vi "SW_Load_data_from_older_TDMS.vi"(4 "Data samples to load":i64=-1, 8 "error in (no error)":errorcluster, 11 "TDMS file ref.":refnum<k34>) -> (0 "error out":errorcluster, 1 "Start time":dbl, 2 "Author's name":string, 3 "Loaded data":T1={"Absolute timestamp (DBL)"=[], "Relative timestamp (DBL)"=[], "Zones normalized allocation array"=[], "Coordinates and speed"=[], "Current zone and TTLs"=[], "Acquisition settings cluster out"={"Researcher name"="", "N segments MIDFIELD"=0, "N segments BORDER"=0, "Radius, mm CENTER"=0, "Radius, mm MIDFIELD"=0, "Starting angle MIDFIELD"=0, "Starting angle BORDER"=0, "Cage diameter, mm"=0, "Bridge swap"=FALSE, "Bridge V. offset"=0.0, "Twisted neck"=FALSE, "Offset H."=0.0, "Name prefix"="SavedTrack", "Stop at"=0.0, "\"Stop at\" enabled"=FALSE, "Settings loaded OK"=FALSE}, "Stimulus presets array"=[]} {"Acquisition settings cluster out"."Stop at" format="%<%H:%M:%S>t"}, 5 "Data loaded OK":bool, 7 "Settings loaded OK":bool)   [LabVIEW 2018, in "Tracker.lvlib"]
uses:
  Tracker.lvlib
panel:
  out "Stimulus presets array (loaded)":T2(array[cluster])
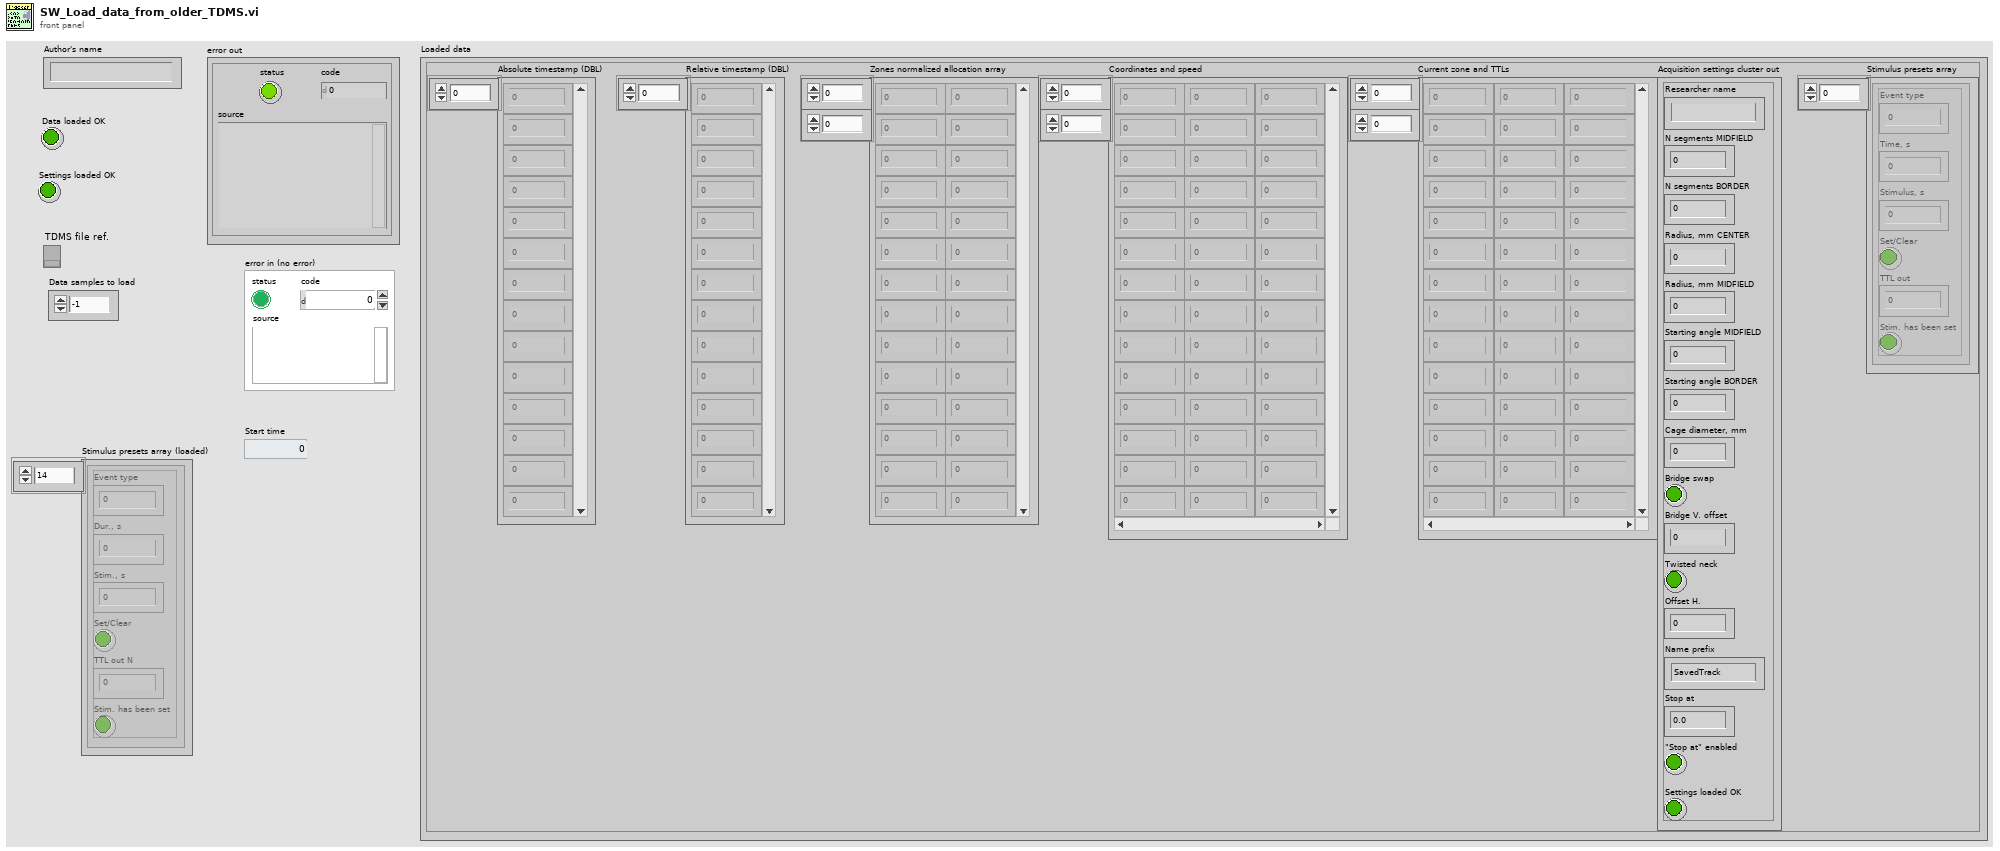
[diagram p1: front panel]
types:
  T1 = cluster{"Absolute timestamp (DBL)":dbl[], "Relative timestamp (DBL)":dbl[], "Zones normalized allocation array":dbl[][], "Coordinates and speed":dbl[][], "Current zone and TTLs":u8[][], "Acquisition settings cluster out":cluster{"Researcher name":string, "N segments MIDFIELD":u8, "N segments BORDER":u8, "Radius, mm CENTER":u16, "Radius, mm MIDFIELD":u16, "Starting angle MIDFIELD":i16, "Starting angle BORDER":i16, "Cage diameter, mm":u16, "Bridge swap":bool, "Bridge V. offset":sgl, "Twisted neck":bool, "Offset H.":sgl, "Name prefix":string, "Stop at":dbl, "\"Stop at\" enabled":bool, "Settings loaded OK":bool}, "Stimulus presets array":cluster{"Event type":u16, "Time, s":sgl, "Stimulus, s":sgl, "Set/Clear":bool, "TTL out":u16, "Stim. has been set":bool}[]}
  T2 = cluster{"Event type":u16, "Dur., s":sgl, "Stim., s":sgl, "Set/Clear":bool, "TTL out N":u16, "Stim. has been set":bool}[]
  T3 = cluster{"N segments BORDER":u8, "Starting angle BORDER":i16, "N segments MIDFIELD":u8, "Starting angle MIDFIELD":i16, "Radius, mm MIDFIELD":u16, "Amount of central segments":u8, "Radius, mm CENTER":u16, "Bridge swap":bool, "Bridge V. offset":sgl, "Twisted neck":bool, "Offset H.":sgl, "Zones configuration":string[], "IO parameters string":string, "Cage diameter, mm":u16, "Name prefix":string, "Stop at":dbl, "\"Stop at\" enabled":bool}
  T4 = cluster{"Event type":u16, "Time, s":sgl, "Stimulus, s":sgl, "Set/Clear":bool, "TTL out":u16, "Stim. has been set":bool}
  T5 = cluster{string, "N segments MIDFIELD":u8, "N segments BORDER":u8, "Radius, mm CENTER":u16, "Radius, mm MIDFIELD":u16, "Starting angle MIDFIELD":i16, "Starting angle BORDER":i16, "Cage diameter, mm":u16, "Bridge swap":bool, "Bridge V. offset":sgl, "Twisted neck":bool, "Offset H.":sgl, "Name prefix":string, "Stop at":dbl, "\"Stop at\" enabled":bool, bool}
  T6 = cluster{dbl[], dbl[], "Zones normalized allocation array":dbl[][], dbl[][], u8[][], cluster{string, "N segments MIDFIELD":u8, "N segments BORDER":u8, "Radius, mm CENTER":u16, "Radius, mm MIDFIELD":u16, "Starting angle MIDFIELD":i16, "Starting angle BORDER":i16, "Cage diameter, mm":u16, "Bridge swap":bool, "Bridge V. offset":sgl, "Twisted neck":bool, "Offset H.":sgl, "Name prefix":string, "Stop at":dbl, "\"Stop at\" enabled":bool, bool}, cluster{"Event type":u16, "Time, s":sgl, "Stimulus, s":sgl, "Set/Clear":bool, "TTL out":u16, "Stim. has been set":bool}[]}
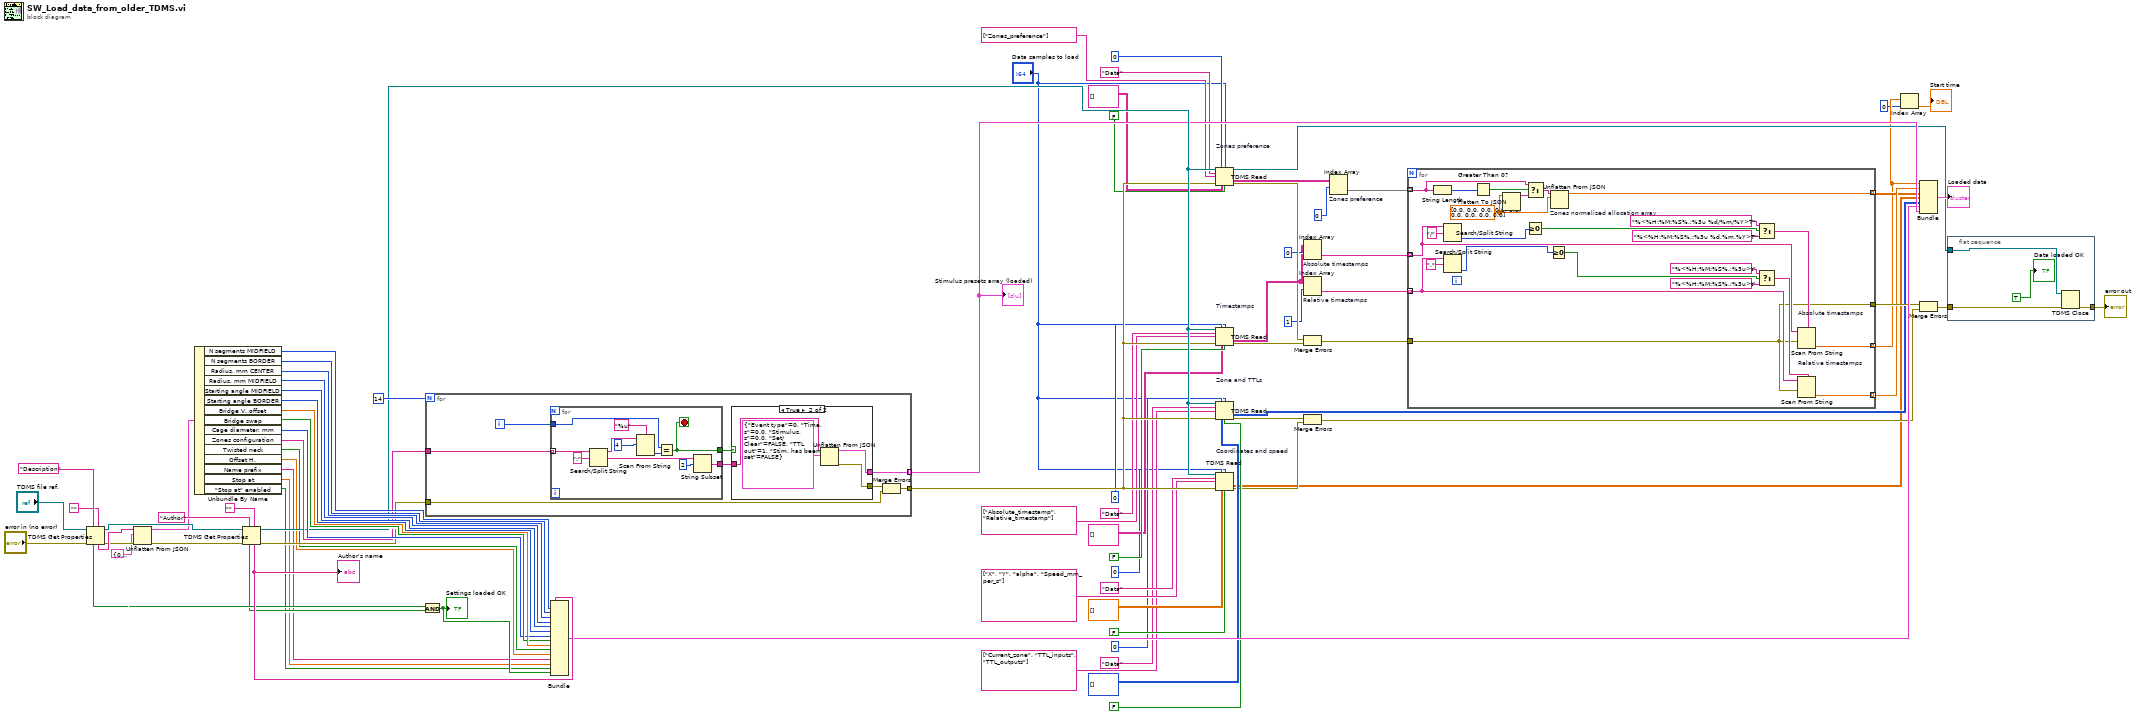
[diagram p0: block diagram]
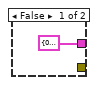
[diagram p2: hidden frame]
diagram:
  n1 = TDMS Get Properties(5:"", 7:"Description" ("property name"), 8:"error in (no error)", 11:"TDMS file ref.") -> (0:w81:errorcluster, 3:w80:refnum<k34>, 4:w82:string, 6:w65:bool)  [unwired: 2 in, 2 out]
  n2 = Unflatten From JSON(JSON string=w82, type and defaults=T3 {"N segments BORDER"=0, "Starting angle BORDER"=0, "N segments MIDFIELD"=0, "Starting angle MIDFIELD"=0, "Radius, mm MIDFIELD"=0, "Amount of central segments"=0, "Radius, mm CENTER"=0, "Bridge swap"=FALSE, "Bridge V. offset"=0.0, "Twisted neck"=FALSE, "Offset H."=0.0, "Zones configuration"=[], "IO parameters string"="[12,1,1,0,0,0]", "Cage diameter, mm"=180, "Name prefix"="SavedTrack", "Stop at"=0.0, "\"Stop at\" enabled"=FALSE} ("Parameters"), error in (no error)=w81) -> (value=w67:T3, error out=w77:errorcluster)  [unwired: 4 in]
  n3 = Unbundle By Name(w67) -> ("N segments MIDFIELD"=w75:u8, "N segments BORDER"=w74:u8, "Radius, mm CENTER"=w73:u16, "Radius, mm MIDFIELD"=w72:u16, "Starting angle MIDFIELD"=w71:i16, "Starting angle BORDER"=w70:i16, "Bridge V. offset"=w69:sgl, "Bridge swap"=w68:bool, "Cage diameter, mm"=w66:u16, "Zones configuration"=w62:string[], "Twisted neck"=w54:bool, "Offset H."=w53:sgl, "Name prefix"=w52:string, "Stop at"=w51:dbl, "\"Stop at\" enabled"=w50:bool)
  n4 = TDMS Get Properties(5:"", 7:"Author" ("property name"), 8:w77, 11:w80) -> (0:w63:errorcluster, 3:w60:refnum<k34>, 4:w76:string, 6:w64:bool)  [unwired: 2 in, 2 out]
  "Author's name" <- w76
  n5 = And(x=w65, y=w64) -> (x .and. y?=w55:bool)
  "Settings loaded OK" <- w55
  n6 = for {
    N: 14 -> [_]
    tunnel: w63 -> [w89]
    tunnel: [w91] -> w59
    tunnel: [w92] -> w58 mode=indexing
    tunnel: w62 -> [w87]
    i -> [w88]
    n7 = for {
      tunnel: w87 -> [w103] mode=indexing
      tunnel: w88 -> [w97]
      tunnel: [w96] -> w86
      tunnel: [w95] -> w85
      stop <- w96 stop-if-true
      n8 = Search/Split String(string=w103, search string/char (-)=":") -> (substring before match=w101:string, match + rest of string=w94:string)  [unwired: 1 in, 1 out]
      n9 = Scan From String(format string="%u", input string=w101, initial scan location=u32 4) -> (output 1=w98:u32)  [unwired: 2 in, 3 out]
      n10 = Equal?(x=w97, y=w98) -> (x = y?=w96:bool)
      n11 = String Subset(string=w94, offset (0)=2) -> (substring=w95:string)  [unwired: 1 in]
    }
    n12 = case shown="True" w86 {
      tunnel: w85 -> [_ w108]
      tunnel: [T4 {"Event type"=0, "Time, s"=0.0, "Stimulus, s"=0.0, "Set/Clear"=FALSE, "TTL out"=1, "Stim. has been set"=FALSE} ("Cluster of the stimuls settings") w107] -> w92
      tunnel: [_ w106] -> w90
      frame False {
      }
      frame True {
        n13 = Unflatten From JSON(JSON string=w108, type and defaults=T4 {"Event type"=0, "Time, s"=0.0, "Stimulus, s"=0.0, "Set/Clear"=FALSE, "TTL out"=1, "Stim. has been set"=FALSE} ("Cluster of the stimuls settings")) -> (value=w107:T4, error out=w106:errorcluster)  [unwired: 5 in]
      }
    }
    n14 = Merge Errors(w90, w89) -> (w91:errorcluster)
  }
  "Stimulus presets array (loaded)" <- w58
  n15 = Bundle(w76, "N segments MIDFIELD"=w75, "N segments BORDER"=w74, "Radius, mm CENTER"=w73, "Radius, mm MIDFIELD"=w72, "Starting angle MIDFIELD"=w71, "Starting angle BORDER"=w70, "Cage diameter, mm"=w66, "Bridge swap"=w68, "Bridge V. offset"=w69, "Twisted neck"=w54, "Offset H."=w53, "Name prefix"=w52, "Stop at"=w51, "\"Stop at\" enabled"=w50, w55) -> (w57:T5)  [unwired: 1 in]
  n16 = TDMS Read "Zones preference"(0:w60, 1:i64 0 ("offset (0)"), 2:"Data samples to load", 5:"Data" ("group name in"), 7:string[] ["Zones_preference"] ("Columns Names"), 11:w59, 12:string[][] [], 13:FALSE ("return channels in file order? (F)")) -> (4:w9:refnum<k34>, 10:w19:string[][], 15:w30:errorcluster)  [unwired: 3 out]
  n17 = TDMS Read "Timestamps"(0:w60, 1:i64 0 ("offset (0)"), 2:"Data samples to load", 5:"Data" ("group name in"), 7:string[] ["Absolute_timestamp", "Relative_timestamp"] ("Columns Names"), 11:w59, 12:string[][] [], 13:FALSE ("return channels in file order? (F)")) -> (10:w23:string[][], 15:w29:errorcluster)  [unwired: 4 out]
  n18 = TDMS Read "Zone and TTLs"(0:w60, 1:i64 0 ("offset (0)"), 2:"Data samples to load", 5:"Data" ("group name in"), 7:string[] ["Current_zone", "TTL_inputs", "TTL_outputs"] ("Columns Names"), 11:w59, 12:u8[][] [], 13:FALSE ("return channels in file order? (F)")) -> (10:w12:u8[][], 15:w28:errorcluster)  [unwired: 4 out]
  n19 = TDMS Read "Coordinates and speed"(0:w60, 1:i64 0 ("offset (0)"), 2:"Data samples to load", 5:"Data" ("group name in"), 7:string[] ["X", "Y", "alpha", "Speed_mm_per_s"] ("Columns Names"), 11:w59, 12:dbl[][] [], 13:FALSE ("return channels in file order? (F)")) -> (10:w11:dbl[][], 15:w17:errorcluster)  [unwired: 4 out]
  n20 = Index Array "Absolute timestamps"(array=w23, index (row)=0) -> (element=w22:string[])  [unwired: 1 in]
  n21 = Index Array "Relative timestamps"(array=w23, index (row)=1) -> (element=w21:string[])  [unwired: 1 in]
  n22 = Merge Errors(w30, w29) -> (w31:errorcluster)
  n23 = Merge Errors(w28, w17) -> (w16:errorcluster)
  n24 = Index Array "Zones preference"(array=w19, index (row)=0) -> (element=w18:string[])  [unwired: 1 in]
  n25 = for {
    tunnel: w31 -> [w109]
    tunnel: [w109] -> w27
    tunnel: w22 -> [w113] mode=indexing
    tunnel: w21 -> [w111] mode=indexing
    tunnel: w18 -> [w115] mode=indexing
    tunnel: [w114] -> w14 mode=indexing
    tunnel: [w112] -> w3 mode=indexing
    tunnel: [w110] -> w15 mode=indexing
    w116 = dbl[] [0.0, 0.0, 0.0, 0.0, 0.0, 0.0, 0.0, 0.0, 0.0] ("Zones normalized allocation array")
    n26 = String Length(string=w115) -> (length=w120:i32)
    n27 = Search/Split String(string=w111, search string/char (-)=".") -> (offset of match=w124:i32)  [unwired: 1 in, 2 out]
    n28 = Search/Split String(string=w113, search string/char (-)="/") -> (offset of match=w128:i32)  [unwired: 1 in, 2 out]
    n29 = Greater Than 0?(x=w120) -> (x > 0?=w119:bool)
    n30 = Flatten To JSON(anything=w116) -> (JSON string=w117:string)  [unwired: 2 in, 1 out]
    n31 = Greater Or Equal To 0?(x=w128) -> (x >= 0?=w127:bool)
    n32 = Select(t=w115, s=w119, f=w117) -> (s? t:f=w118:string)
    n33 = Greater Or Equal To 0?(x=w124) -> (x >= 0?=w121:bool)
    n34 = Unflatten From JSON "Zones normalized allocation array"(JSON string=w118, type and defaults=w116) -> (value=w114:dbl[])  [unwired: 5 in, 1 out]
    n35 = Select(t="%<%H:%M:%S%.;%3u %d/%m/%Y>T" ("format string"), s=w127, f="%<%H:%M:%S%,;%3u %d.%m.%Y>T" ("format string")) -> (s? t:f=w130:string)
    n36 = Select(t="%<%H:%M:%S%.;%3u>t" ("format string"), s=w121, f="%<%H:%M:%S%,;%3u>t" ("format string")) -> (s? t:f=w126:string)
    n37 = Scan From String "Absolute timestamps"(format string=w130, input string=w113, error in=w109) -> (output 1=w112:dbl)  [unwired: 2 in, 3 out]
    n38 = Scan From String "Relative timestamps"(format string=w126, input string=w111, error in=w109) -> (output 1=w110:dbl)  [unwired: 2 in, 3 out]
  }
  n39 = Index Array(array=w3, index=0) -> (element=→"Start time":dbl)
  n40 = Bundle(w3, w15, "Zones normalized allocation array"=w14, w11, w12, w57, w58) -> (→"Loaded data":T6)  [unwired: 1 in]
  n41 = Merge Errors(w27, w16) -> (w26:errorcluster)
  n42 = flat-sequence {
    tunnel: [w135] -> w10
    tunnel: w26 -> [w133]
    tunnel: w9 -> [w134]
    frame #0 {
      n43 = TDMS Close(8:w133, 11:w134) -> (0:w135:errorcluster)  [unwired: 1 out]
      "Data loaded OK" <- TRUE ("notification")
    }
  }
  "error out" <- w10
